vi "Set Multi Gate Hysteresis [HMS].vi"(6 "Gate Number":i32, 7 "Micropulse # In":i32, 8 "error in (no error)":errorcluster, 9 "Hysteresis":T1, 11 "Test Number":u32) -> (0 "error out":errorcluster, 5 "Micropulse # Out":i32)   [LabVIEW 2026, in "MicroPulse_Driver.lvlib"]
doc: "Multi-gate version of HYS command. The hysteresis function governs whether secondary peaks are reported as separated indications or not and works by assigning a value in dB that the signal must fall before the half cycle is considered as a separate meaningful signal. Conversely, following a peak validation the system tracks and validates the trough using the same value.\n\nParameters:\n<Tn> : Test number. An integer value from 0 to the maximum number of tests (default maximum is 1279 tests).\nTn = 0 for all conventional tests. If the S extension is used it applies to all tests in the sweep number specified: 1-32, 0 = all sweeps.\n\n<Gn> : Gate Number, an integer value from 0 to 4.\nGn = 0 for all gates in the test\n\n<Hysteresis level> : \n0 = No Hysteresis\n1 = 3dB\n2 = 6dB (Default level)\n3 = 9dB\n4 =12dB\n\nNote 1: Valid in Multi-gate Mode only (AMP 31 & 32)"
uses:
  MicroPulse_Driver.lvlib
  Data/Datatypes/MP - hysteresis level.ctl
  Private/MP-Registry Action-Enum.ctl
  <instrlib>/Micropulse/Micropulse.lvlib
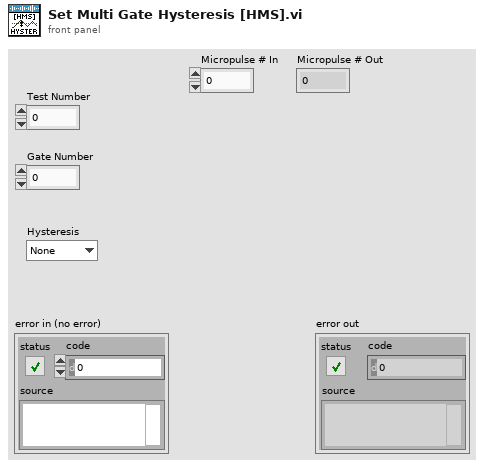
[diagram p1: front panel]
types:
  T1 = typedef "Micropulse.lvlib/MP - hysteresis level.ctl" = enum16{"None", "3dB", "6dB", "9dB", "12dB"}
  T2 = typedef "MicroPulse_Driver.lvlib/MP-Registry Action-Enum.ctl" = enum16{"Read", "Add Test", "Add Command", "Add Gate Command", "Add Encoder Command", "Clear Command  List", "Set Registry", "Set System Details", "Set DOF", "Set Velocity", "Disable Asynch Reads", "Enable Asynch Reads", "Add Connection", "Disconnect", "Shutdown"}
  T3 = typedef "Micropulse.lvlib/TCP config.ctl" = cluster{"Connection ID":refnum<k5>, "IP address":string, "host port":u16, "OC timeout":i32, "Read timeout":i32, "Write timeout":i32}
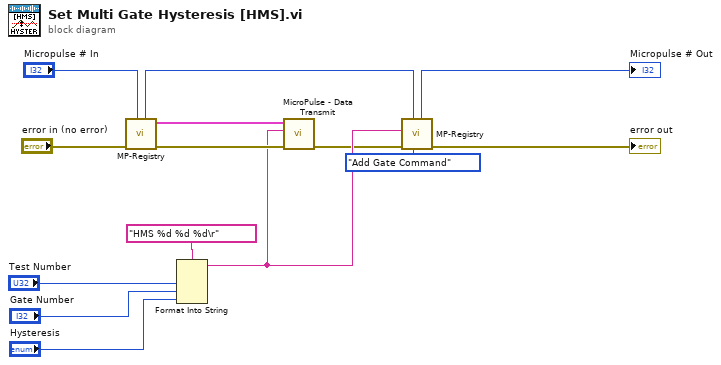
[diagram p0: block diagram]
diagram:
  n1 = call "MP-Registry.vi"("Micropulse # In"="Micropulse # In", "error in (no error)"="error in (no error)") -> ("error out"=w12:errorcluster, "TCP config"=w11:T3, "Micropulse # Out"=w5:i32)  [unwired: 6 in, 1 out]
  n2 = Format Into String(format string="HMS %d %d %d\r", "Test Number", "Gate Number", "Hysteresis") -> (resulting string=w9:string)  [unwired: 2 in, 1 out]
  n3 = call "MicroPulse - Data Transmit.vi"("error in (no error)"=w12, "data"=w9, "TCP config"=w11) -> ("error out"=w7:errorcluster)  [unwired: 6 in, 2 out]
  n4 = call "MP-Registry.vi"("Action"=MP-Registry_Action-Enum."Add Gate Command", "Micropulse # In"=w5, "error in (no error)"=w7, "Data in"=w9) -> ("error out"=→"error out":errorcluster, "Micropulse # Out"=→"Micropulse # Out":i32)  [unwired: 4 in, 2 out]
